vi "Validate Fixed Header.vi"(8 "error in (no error)":errorcluster, 11 "ControlPacket in":refnum<class "ControlPacket.lvclass">) -> (0 "error out":errorcluster, 1 "Valid":bool, 3 "ControlPacket out":refnum<class "ControlPacket.lvclass">)   [LabVIEW 2013, in "ControlPacket.lvclass"]
uses:
  ControlPacket.lvclass
  ControlPacket.lvclass/ControlPacket.ctl
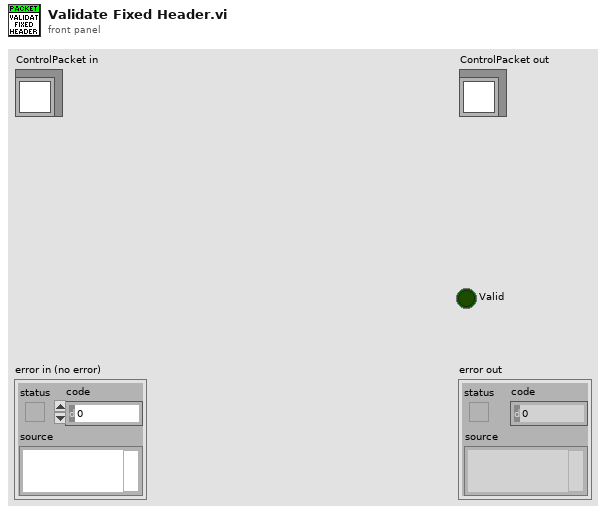
[diagram p1: front panel]
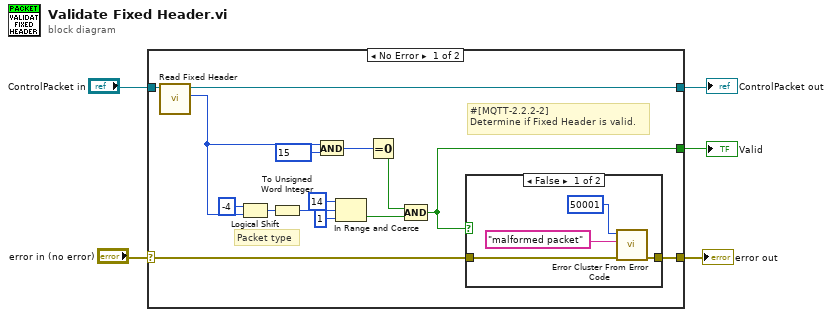
[diagram p0: block diagram]
diagram:
  n1 = case shown="No Error" "error in (no error)" {
    selector: "error in (no error)" -> [w17 w27]
    tunnel: [w16 w27] -> w4
    tunnel: [w6 _] -> w1
    tunnel: [w20 w26] -> w2
    tunnel: "ControlPacket in" -> [w18 w26]
    frame No Error {
      # "#[MQTT-2.2.2-2]\nDetermine if Fixed Header is valid."
      # "Packet type"
      n2 = call "Read Fixed Header.vi"("ControlPacket in"=w18) -> ("Fixed Header"=w9:u8, "ControlPacket out"=w20:refnum<class "ControlPacket.lvclass">)  [unwired: 9 in]
      n3 = Logical Shift(y=i16 -4, x=w9) -> (x << y=w11:u8)
      n4 = To Unsigned Word Integer(number=w11) -> (unsigned 16bit integer=w10:u16)
      n5 = And(x=w9, y=u8 15) -> (x .and. y?=w15:u8)
      n6 = In Range and Coerce(upper limit=u16 14, x=w10, lower limit=u16 1) -> (In Range?=w8:bool)  [unwired: 1 out]
      n7 = Equal To 0?(x=w15) -> (x = 0?=w7:bool)
      n8 = Compound Arithmetic op=AND(w7, w8) -> (w6:bool)
      n9 = case shown="False" w6 {
        tunnel: [w22 w25] -> w16
        tunnel: w17 -> [w21 w25]
        frame False {
          n10 = call <vilib>:"Error Cluster From Error Code.vi"("error in (no error)"=w21, "error message (\"\")"="malformed packet" ("error message (\"\")"), "error code (0)"=50001) -> ("error out"=w22:errorcluster)  [unwired: 6 in]
        }
        frame True {
        }
      }
    }
    frame Error {
    }
  }
  "Valid" <- w1
  "error out" <- w4
  "ControlPacket out" <- w2
